vi "配置初始化.vi"(8 "error in (no error)":errorcluster caption="错误输入（无错误）") -> (0 "错误输出":errorcluster)   [LabVIEW 2022 SP3, in "流量计集成.lvlib"]
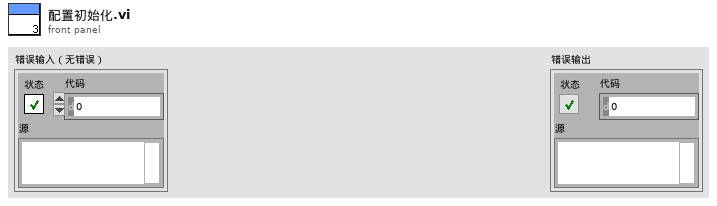
[diagram p1: front panel]
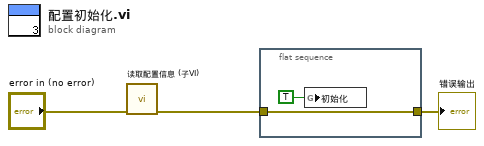
[diagram p0: block diagram]
diagram:
  n1 = call "读取配置信息 (子VI).vi"("error in (no error)"="error in (no error)") -> ("错误输出"=w2:errorcluster)  [unwired: 10 in]
  n2 = flat-sequence {
    tunnel: [w4] -> w1
    tunnel: w2 -> [w4]
    frame #0 {
      n3 = global write "流量计全局变量.vi" "初始化"(TRUE ("初始化")) -> ()
    }
  }
  "错误输出" <- w1
